vi "Do.vi"(8 "error in (no error)":errorcluster, 10 "Actor in":refnum<class "Actor.lvclass">, 11 "Read QDEvent Logfile Msg":refnum<class "Read QDEvent Logfile Msg.lvclass">) -> (0 "error out":errorcluster, 2 "Actor out":refnum<class "Actor.lvclass">)   [LabVIEW 2016, in "KIT-QA.lvlib" / "Read QDEvent Logfile Msg.lvclass"]
doc: "This VI delivers the message to the actor by calling the appropriate method(s) on the actor."
uses:
  Read QDEvent Logfile Msg.lvclass
  <vilib>/ActorFramework/Actor/Actor.lvclass
  KIT-QA/KIT-QA.lvclass
  C:/Program Files (x86)/National Instruments/LabVIEW 2016/vi.lib/ActorFramework/Actor/Actor.lvclass
  Read QDEvent Logfile Msg.lvclass/Read QDEvent Logfile Msg.ctl
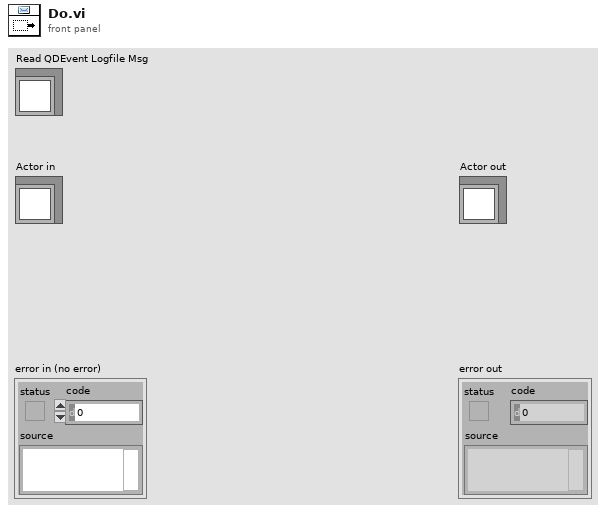
[diagram p1: front panel]
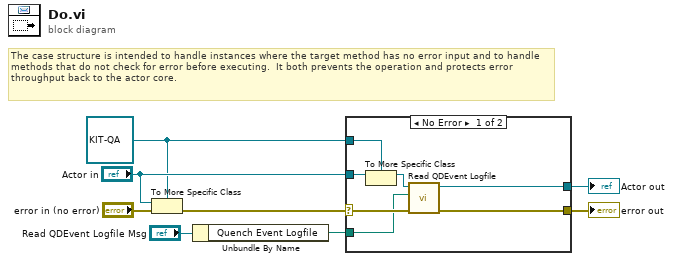
[diagram p0: block diagram]
diagram:
  w3 = refnum<class "KIT-QA.lvclass"> refnum ("Actor in")
  # "The case structure is intended to handle instances where the target method has no error input and to handle methods that do not check for error before executing.  It both prevents the operation and protects error throughput back to the actor core."
  n1 = To More Specific Class(target class=w3, reference="Actor in", error in="error in (no error)") -> (error out=w7:errorcluster)  [unwired: 1 out]
  n2 = Unbundle By Name("Read QDEvent Logfile Msg") -> ("Quench Event Logfile"=w1:path)
  n3 = case shown="No Error" w7 {
    selector: w7 -> [w13 w17]
    tunnel: [w15 w17] -> w6
    tunnel: [w14 w16] -> w5
    tunnel: "Actor in" -> [w12 w16]
    tunnel: w3 -> [w11 _]
    tunnel: w1 -> [w9 _]
    frame No Error {
      n4 = To More Specific Class(target class=w11, reference=w12) -> (specific class reference=w10:refnum<class "KIT-QA.lvclass">)  [unwired: 1 in, 1 out]
      n5 = call "Read QDEvent Logfile.vi"("Error In"=w13, "Quench Event Logfile"=w9, "KIT-QA in"=w10) -> ("Error Out"=w15:errorcluster, "KIT-QA out"=w14:refnum<class "KIT-QA.lvclass">)  [unwired: 7 in]
    }
    frame Error {
      # "If type check fails, pass the original object out again."
    }
  }
  "error out" <- w6
  "Actor out" <- w5
